vi "PH_GUI.set picture GUI object.vi"(0 "Visible (true)":bool=TRUE, 2 "CtlRef":refnum<vi>, 3 "Picture":picture, 4 "Tip Strip (\"\")":string, 5 "error in (no error)":errorcluster) -> (19 "error out":errorcluster)   [LabVIEW 2014, in "PH_Common.lvlib"]
doc: "Sets value and more for the referenced GUI object."
uses:
  PH_Common.lvlib
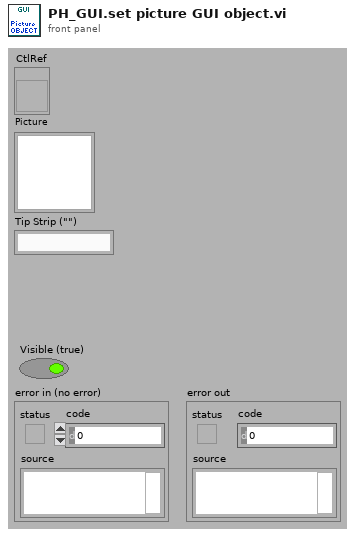
[diagram p1: front panel]
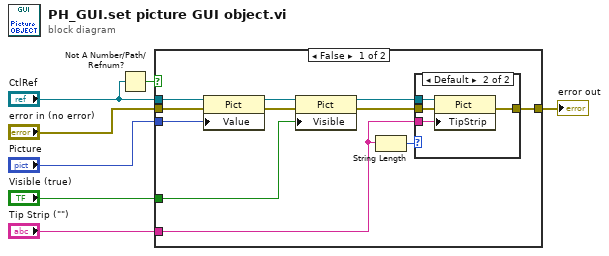
[diagram p0: block diagram]
diagram:
  n1 = Not A Number/Path/Refnum?(number/path/refnum="CtlRef") -> (NaN/Path/Refnum?=w6:bool)
  n2 = case shown="False" w6 {
    tunnel: [w15 w24] -> w2
    tunnel: "CtlRef" -> [w18 _]
    tunnel: "error in (no error)" -> [w17 w24]
    tunnel: "Tip Strip (\"\")" -> [w13 _]
    tunnel: "Picture" -> [w16 _]
    tunnel: "Visible (true)" -> [w12 _]
    frame False {
      n3 = property class="Pict"(reference=w18, error in=w17, "Value"=w16) -> (reference out=w11:refnum<vi>, error out=w10:errorcluster)
      n4 = property class="Pict"(reference=w11, error in=w10, "Visible"=w12) -> (reference out=w9:refnum<vi>, error out=w8:errorcluster)
      n5 = String Length(string=w13) -> (length=w14:i32)
      n6 = case shown="Default" w14 {
        tunnel: w8 -> [w19 w23]
        tunnel: [w19 w22] -> w15
        tunnel: w9 -> [_ w21]
        tunnel: w13 -> [_ w20]
        frame 0 {
        }
        frame Default {
          n7 = property class="Pict"(reference=w21, error in=w23, "TipStrip"=w20) -> (error out=w22:errorcluster)  [unwired: 1 out]
        }
      }
    }
    frame True {
    }
  }
  "error out" <- w2
